vi "Create Scheduled Gap.vi"(8 "error in":errorcluster, 11 "1553 Scheduled Message Configuration in":T1) -> (0 "error out":errorcluster, 3 "gap item out":refnum<k24>)   [LabVIEW 2020, in "Ballard_1553_Hardware_ni.lvlib"]
uses:
  Ballard_1553_Hardware_ni.lvlib
  C:/Users/Administrator/Desktop/GIT/Ballard-MIL-STD-1553-Custom-Device/Source/System Explorer/SubVIs/Parse XML Ballard/1.2/BTIXML_SerDes.dll
  Ballard-MIL-STD-1553-Custom-Device/Source/System Explorer/SubVIs/Parse XML Ballard/1.2/BTIXML_SerDes.dll
  _typedefs/schedItem1553_type.ctl
  _typedefs/frame_entry_type.ctl
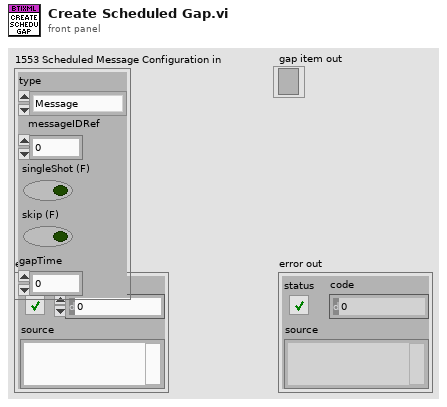
[diagram p1: front panel]
types:
  T1 = typedef "Ballard_1553_Hardware_ni.lvlib/schedItem1553_type.ctl" = cluster{"type":T2, "messageIDRef":i32, "singleShot (F)":bool, "skip (F)":bool, "gapTime":dbl}
  T2 = typedef "Ballard_1553_Hardware_ni.lvlib/frame_entry_type.ctl" = enum16{"Message", "Gap", "Pulse", "Log", "Pause", "Restart", "Halt"}
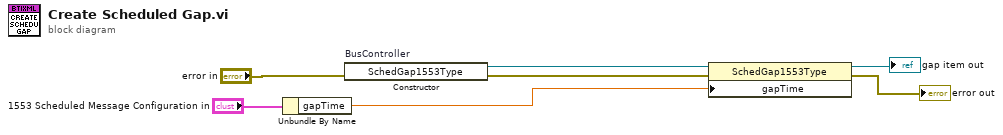
[diagram p0: block diagram]
diagram:
  n1 = Unbundle By Name("1553 Scheduled Message Configuration in") -> ("gapTime"=w2:dbl)
  n2 = constructor on="BusController" class="SchedGap1553Type"(error in="error in") -> (reference out=w6:refnum<k24>, error out=w5:errorcluster)  [unwired: 2 in, 1 out]
  n3 = property class="SchedGap1553Type"(reference=w6, error in=w5, "gapTime"=w2) -> (reference out=→"gap item out":refnum<k24>, error out=→"error out":errorcluster)
